vi "Read Output.vi"(8 "error in (no error)":errorcluster, 11 "VISA resource name":refnum<visa-resource-name>) -> (0 "error out":errorcluster, 1 "Actual Current Level (A)":dbl format="%.3f", 2 "Actual Voltage Level (V)":dbl format="%.3f", 3 "VISA resource name out":refnum<visa-resource-name>, 4 "Read V":string, 6 "Read I":string)   [LabVIEW 2020]
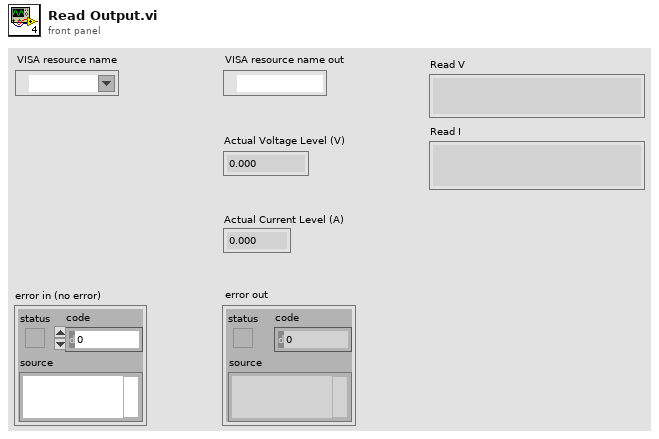
[diagram p1: front panel]
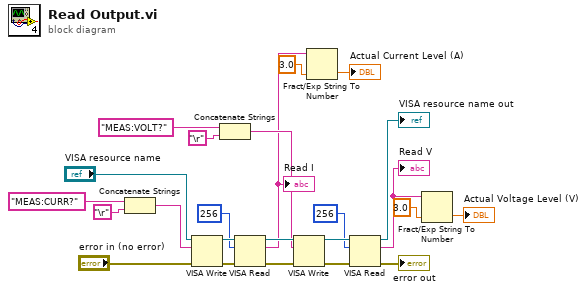
[diagram p0: block diagram]
diagram:
  n1 = Concatenate Strings("MEAS:CURR?" ("write buffer"), "\r") -> (w10:string)
  n2 = VISA Write(VISA resource name="VISA resource name", write buffer=w10, error in (no error)="error in (no error)") -> (VISA resource name out=w14:refnum<visa-resource-name>, error out=w15:errorcluster)  [unwired: 1 out]
  n3 = Concatenate Strings("MEAS:VOLT?" ("write buffer"), "\r") -> (w18:string)
  n4 = VISA Read(VISA resource name=w14, byte count=u32 256, error in (no error)=w15) -> (VISA resource name out=w23:refnum<visa-resource-name>, read buffer=w8:string, error out=w2:errorcluster)  [unwired: 1 out]
  "Read I" <- w8
  n5 = VISA Write(VISA resource name=w23, write buffer=w18, error in (no error)=w2) -> (VISA resource name out=w24:refnum<visa-resource-name>, error out=w22:errorcluster)  [unwired: 1 out]
  n6 = Fract/Exp String To Number(string=w8, default (0 dbl)=3.0 ("valeur par défaut (0 DBL)")) -> (number=→"Actual Current Level (A)":dbl)  [unwired: 2 in, 1 out]
  n7 = VISA Read(VISA resource name=w24, byte count=u32 256, error in (no error)=w22) -> (VISA resource name out=→"VISA resource name out":refnum<visa-resource-name>, read buffer=w5:string, error out=→"error out":errorcluster)  [unwired: 1 out]
  "Read V" <- w5
  n8 = Fract/Exp String To Number(string=w5, default (0 dbl)=3.0 ("valeur par défaut (0 DBL)")) -> (number=→"Actual Voltage Level (V)":dbl)  [unwired: 2 in, 1 out]
